vi "lua_newstate.vi"(8 "error in (no error)":errorcluster, 9 "ud_p":u64, 10 "lua_Alloc_f":u64) -> (0 "error out":errorcluster, 3 "lua_state_p":u64)   [LabVIEW 2020, in "lua.dll.lvlib"]
uses:
  lua.dll.lvlib
  lua54.dll
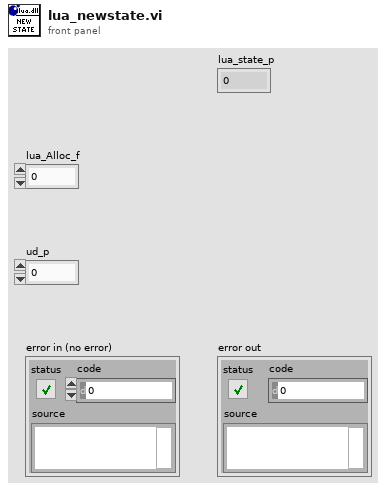
[diagram p1: front panel]
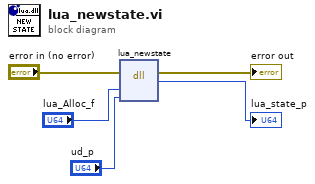
[diagram p0: block diagram]
diagram:
  n1 = dll-call lib="C:/Users/Nicholas Folse/Documents/workspace/github-tauterra.llc/Lua for LabVIEW/lib/lua.dll/lua54**.*" fn="lua_newstate"(error in="error in (no error)", "lua_Alloc_f"="lua_Alloc_f", "ud_p"="ud_p") -> (error out=→"error out":errorcluster, "lua_state_p"=→"lua_state_p":u64)  [unwired: 4 in, 1 out]
